vi "StartVITester.vi"(8 "error in (no error)":errorcluster, 11 "CommandLine":string[](array[string])) -> (0 "error out":errorcluster, 2 "test details":string, 3 "output to action":string)   [LabVIEW 2019]
uses:
  <vilib>/addons/_JKI Toolkits/VI Tester/VI Tester API.llb/Run Tests (Path).vi
  <vilib>/addons/_JKI Toolkits/VI Tester/VI Tester API.llb/VI Tester API.lvlib
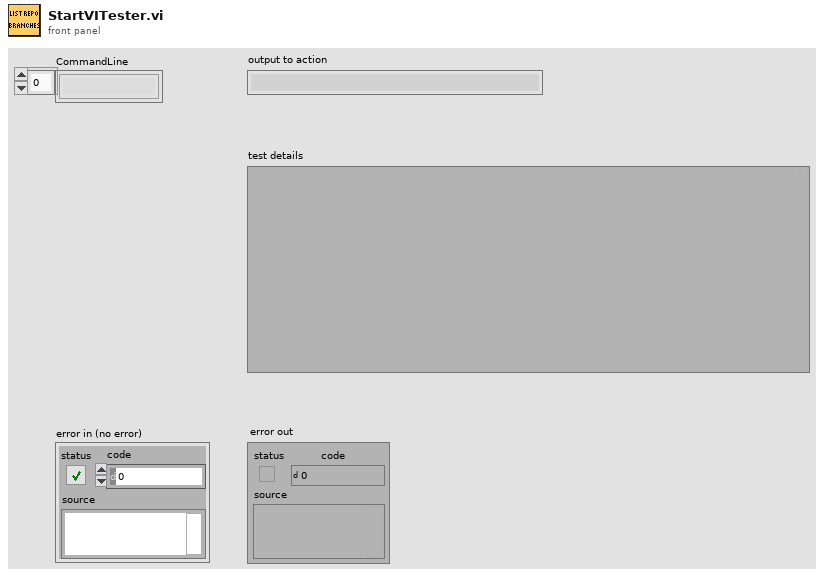
[diagram p1: front panel]
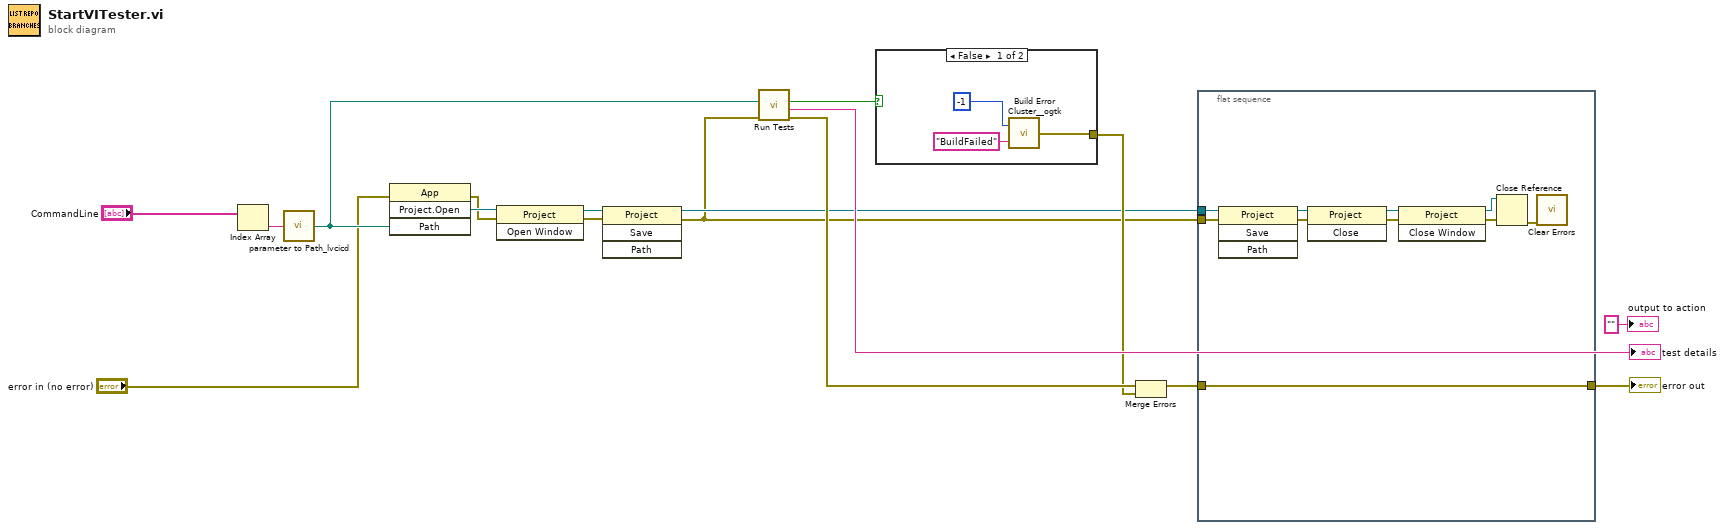
[diagram p0: block diagram]
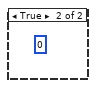
[diagram p2: hidden frame]
diagram:
  n1 = Index Array(array="CommandLine") -> (element=w15:string)  [unwired: 1 in]
  n2 = call "parameter to Path_lvcicd.vi"("String"=w15) -> ("Path"=w17:path)
  n3 = invoke class="App" method="Project.Open"(error in="error in (no error)", "Path"=w17) -> (error out=w10:errorcluster, "Project:Open"=w13:refnum<vi>)  [unwired: 2 in, 2 out]
  n4 = invoke class="Project" method="Open Window"(reference=w13, error in=w10) -> (reference out=w12:refnum<vi>, error out=w11:errorcluster)  [unwired: 1 in, 1 out]
  n5 = invoke class="Project" method="Save"(reference=w12, error in=w11) -> (reference out=w5:refnum<vi>, error out=w4:errorcluster)  [unwired: 2 in, 2 out]
  n6 = call-poly <vilib>:"Run Tests.vi"("error in (no error)"=w4, "Test Path"=w17) -> ("error out"=w7:errorcluster, "test details"=→"test details":string, "successful?"=w14:bool)  [unwired: 7 in]
  n7 = case shown="False" w14 {
    tunnel: [w18 _] -> w6
    frame False {
      n8 = call <userlib>:"Build Error Cluster__ogtk.vi"("String to Prepend to source (\"\")"="BuildFailed" ("String to Prepend to source (\"\")"), "code"=-1) -> ("error out"=w18:errorcluster)
    }
    frame True {
      (unwired) 0
    }
  }
  n9 = Merge Errors(w7, w6) -> (w3:errorcluster)
  n10 = flat-sequence {
    tunnel: w5 -> [w30]
    tunnel: w4 -> [w29]
    tunnel: w3 -> [w21]
    tunnel: [w21] -> w2
    frame #0 {
      n11 = invoke class="Project" method="Save"(reference=w30, error in=w29) -> (reference out=w25:refnum<vi>, error out=w26:errorcluster)  [unwired: 2 in, 2 out]
      n12 = invoke class="Project" method="Close"(reference=w25, error in=w26) -> (reference out=w28:refnum<vi>, error out=w27:errorcluster)  [unwired: 1 in, 1 out]
      n13 = invoke class="Project" method="Close Window"(reference=w28, error in=w27) -> (reference out=w23:refnum<vi>, error out=w24:errorcluster)  [unwired: 1 in, 1 out]
      n14 = Close Reference(reference=w23, error in (no error)=w24) -> (error out=w22:errorcluster)
      n15 = call <vilib>:"Clear Errors.vi"("error in (no error)"=w22) -> ()  [unwired: 5 in, 2 out]
    }
  }
  "error out" <- w2
  "output to action" <- "" ("output to action")
